vi "Ex. 3 While loop application.vi"() -> ()   [LabVIEW 2024]
panel:
  out "Iteration count":i32
  in  "Stop":bool
  out "a-b":dbl
  out "a+b":dbl
  in  "a":dbl
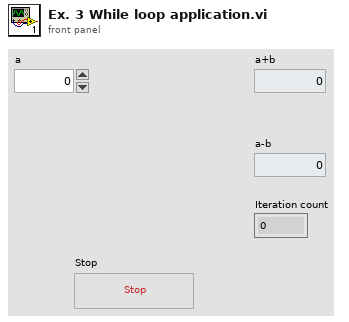
[diagram p1: front panel]
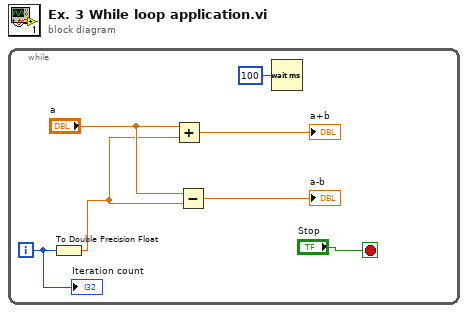
[diagram p0: block diagram]
diagram:
  n1 = while {
    i -> [w3]
    stop <- "Stop" stop-if-true
    n2 = To Double Precision Float(number=w3) -> (double precision float=w2:dbl)
    n3 = Add(x="a", y=w2) -> (x+y=→"a+b":dbl)
    n4 = Subtract(x="a", y=w2) -> (x-y=→"a-b":dbl)
    n5 = Wait (ms)(milliseconds to wait=u32 100) -> ()  [unwired: 1 out]
    "Iteration count" <- w3
  }
